vi "edtFTPnet_Check Folder Exist.vi"(8 "error in(no error)":errorcluster, 10 "remote folder path":path, 11 "FTPClient in":T1) -> (0 "error out":errorcluster, 3 "FTPClient out":T1)   [LabVIEW 2013, in "edtFTPnet.lvlib"]
uses:
  edtFTPnet.lvlib
  Ctrls/edtFTPnet_Session.ctl
  edtFTPnet.dll
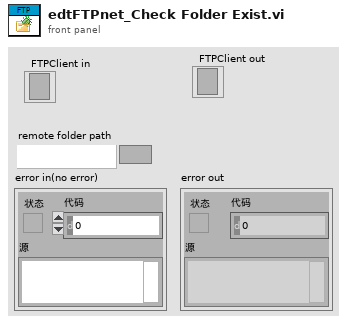
[diagram p1: front panel]
types:
  T1 = typedef "edtFTPnet.lvlib/edtFTPnet_Session.ctl" = refnum<k24>
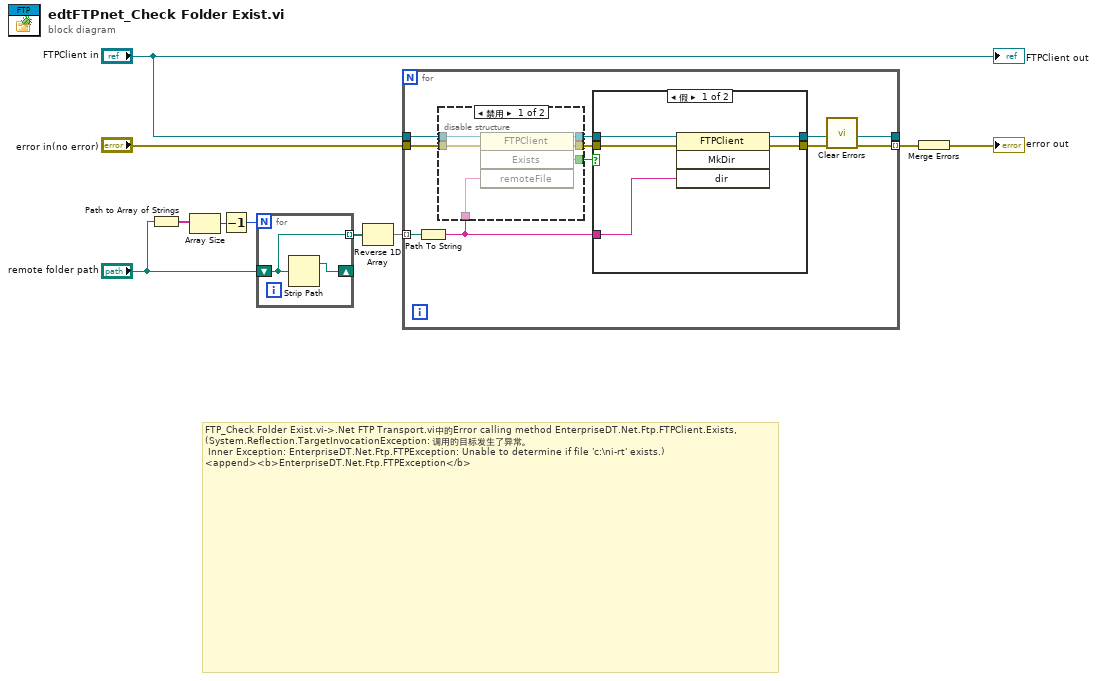
[diagram p0: block diagram]
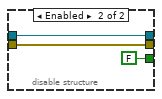
[diagram p2: hidden frame]
diagram:
  # "FTP_Check Folder Exist.vi->.Net FTP Transport.vi中的Error calling method EnterpriseDT.Net.Ftp.FTPClient.Exists, (System.Reflection.TargetInvocationException: 调用的目标发生了异常。\n\tInner Exception: EnterpriseDT.Net.Ftp.FTPException: Unable to determine if file 'c:\\ni-rt' exists.) <append><b>EnterpriseDT.Net.Ftp.FTPException</b>"
  n1 = Path to Array of Strings(0:"remote folder path") -> (2:w6:string[])  [unwired: 1 out]
  n2 = Array Size(array=w6) -> (size(s)=w5:i32)
  n3 = Decrement(x=w5) -> (x-1=w3:i32)
  n4 = for {
    N: w3 -> [_]
    shift-right: [w12] -> _
    shift-left: "remote folder path" -> [w11]
    tunnel: [w11] -> w2 mode=indexing
    n5 = Strip Path(path=w11) -> (stripped path=w12:path)  [unwired: 1 out]
  }
  n6 = Reverse 1D Array(array=w2) -> (reversed array=w4:path[])
  n7 = for {
    tunnel: [w15] -> w7 mode=indexing
    tunnel: "error in(no error)" -> [w22]
    tunnel: "FTPClient in" -> [w21]
    tunnel: [w17] -> _
    tunnel: w4 -> [w20] mode=indexing
    n8 = Path To String(path=w20) -> (string=w14:string)
    n9 = disable-structure shown="禁用" {
      disable-tunnel: w22 -> [w28 w30]
      disable-tunnel: w21 -> [w27 w31]
      disable-tunnel: [w26 w31] -> w19
      disable-tunnel: [w25 w30] -> w18
      disable-tunnel: w14 -> [w24 _]
      disable-tunnel: [w23 FALSE ("Exists")] -> w13
      frame Disabled {
        n10 = invoke class="FTPClient" method="Exists"(reference=w27, error in=w28, "remoteFile"=w24) -> (reference out=w26:T1, error out=w25:errorcluster, "Exists"=w23:bool)  [unwired: 1 in, 1 out]
      }
      frame Enabled {
      }
    }
    n11 = case shown="假" w13 {
      tunnel: w19 -> [w35 w38]
      tunnel: w18 -> [w36 w37]
      tunnel: [w32 w38] -> w17
      tunnel: [w33 w37] -> w16
      tunnel: w14 -> [w34 _]
      frame False {
        n12 = invoke class="FTPClient" method="MkDir"(reference=w35, error in=w36, "dir"=w34) -> (reference out=w32:T1, error out=w33:errorcluster)  [unwired: 1 in, 2 out]
      }
      frame True {
      }
    }
    n13 = call <vilib>:"Clear Errors.vi"("error in (no error)"=w16) -> ("error out"=w15:errorcluster)  [unwired: 6 in]
  }
  n14 = Merge Errors(w7) -> (→"error out":errorcluster)
  "FTPClient out" <- "FTPClient in"
